vi "GetAlarms.vi"(0 "AnalogComparator in":refnum<class "AnalogComparator.lvclass">, 11 "error in (no error)":errorcluster) -> (4 "AnalogComparator out":refnum<class "AnalogComparator.lvclass">, 6 "Alarm":bool, 8 "Warning":bool, 15 "error out":errorcluster)   [LabVIEW 2019, in "AnalogComparator.lvclass"]
uses:
  AnalogComparator.lvclass
  AnalogComparator.lvclass/AnalogComparator.ctl
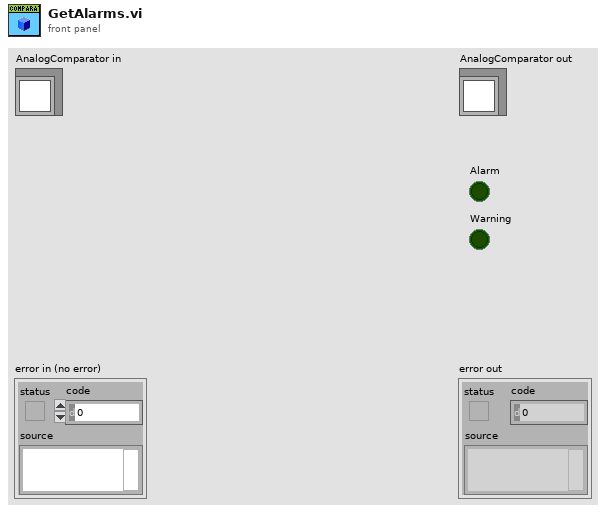
[diagram p1: front panel]
types:
  T1 = typedef "AlarmType.ctl" = enum16{"Normal", "Warning", "Alarm"}
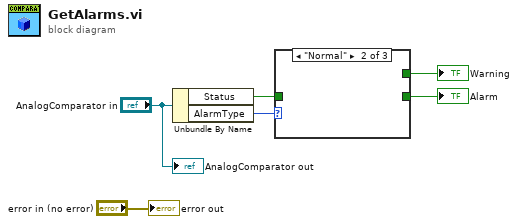
[diagram p0: block diagram]
diagram:
  n1 = Unbundle By Name("AnalogComparator in") -> ("Status"=w2:bool, "AlarmType"=w4:T1)
  n2 = case shown="\"Normal\"" w4 {
    tunnel: [_ _ w8] -> w3
    tunnel: w2 -> [w7 _ w8]
    tunnel: [w7 _ _] -> w1
    frame "Alarm" {
    }
    frame "Normal" {
    }
    frame "Warning" {
    }
  }
  "Alarm" <- w1
  "Warning" <- w3
  "error out" <- "error in (no error)"
  "AnalogComparator out" <- "AnalogComparator in"
